vi "MTM2_putSample_targetForces.vi"(8 "error in (no error)":errorcluster, 11 "targetForces_Ctl":T1) -> (0 "error out":errorcluster, 2 "function return":i32, 3 "targetForces_Ctl out":T1)   [LabVIEW 2018, in "SALLV_MTM2.lvlib"]
doc: "int MTM2_shm_putSample_targetForcesLV(MTM2_targetForcesLV *targetForces_Ctl );"
uses:
  SALLV_MTM2.lvlib
  DataTypes/targetForces.ctl
  SALLV_MTM2.so
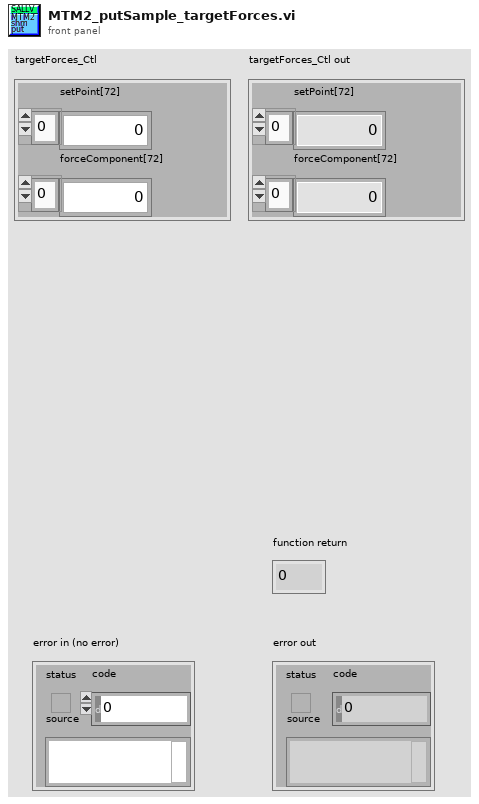
[diagram p1: front panel]
types:
  T1 = typedef "SALLV_MTM2.lvlib/targetForces.ctl" = cluster{"setPoint[72]":dbl[], "forceComponent[72]":dbl[]}
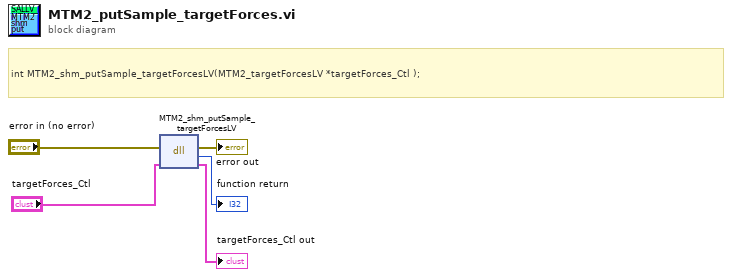
[diagram p0: block diagram]
diagram:
  # "int MTM2_shm_putSample_targetForcesLV(MTM2_targetForcesLV *targetForces_Ctl );"
  n1 = dll-call lib="home/ttsai/Document/salApiMTM2/SALLV_MTM2/SALLV_MTM2.*" fn="MTM2_shm_putSample_targetForcesLV"(error in="error in (no error)", "targetForces_Ctl"="targetForces_Ctl") -> (error out=→"error out":errorcluster, →"function return":i32, "targetForces_Ctl"=→"targetForces_Ctl out":T1)  [unwired: 2 in, 1 out]
